vi "Circular Add (SubVI).vi"(8 "Sum In":u16, 11 "Max. Sum":u16) -> (0 "Sum Out":u16)   [LabVIEW 2015]
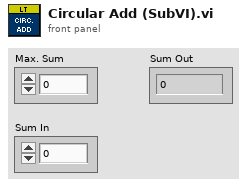
[diagram p1: front panel]
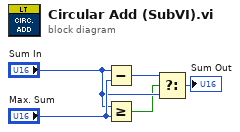
[diagram p0: block diagram]
diagram:
  n1 = Subtract(x="Sum In", y="Max. Sum") -> (x-y=w2:u16)
  n2 = Greater Or Equal?(x="Sum In", y="Max. Sum") -> (x >= y?=w1:bool)
  n3 = Select(t=w2, s=w1, f="Sum In") -> (s? t:f=→"Sum Out":u16)
